vi "FMDemo2 (SubVI).vi"(9 "Numeric":dbl, 10 "Array":cdb[](array[numeric]), 11 "Sample Rate":dbl) -> (3 "Decimated Array":dbl[](array[numeric]))   [LabVIEW 2013]
uses:
  <vilib>/Analysis/3filter.llb/Filter Passband Type.ctl
  <vilib>/Analysis/3filter.llb/Butterworth Filter (CDB).vi
  <vilib>/Analysis/2dsp.llb/Decimate (continuous, DBL).vi
  <vilib>/Analysis/NI_AALBase.lvlib
  <vilib>/Analysis/NI_AALPro.lvlib
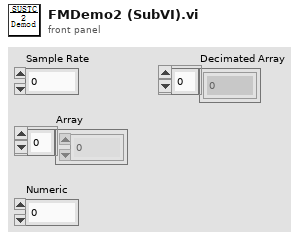
[diagram p1: front panel]
types:
  T1 = typedef "NI_AALBase.lvlib/Filter Passband Type.ctl" = enum32{"Lowpass", "Highpass", "Bandpass", "Bandstop"}
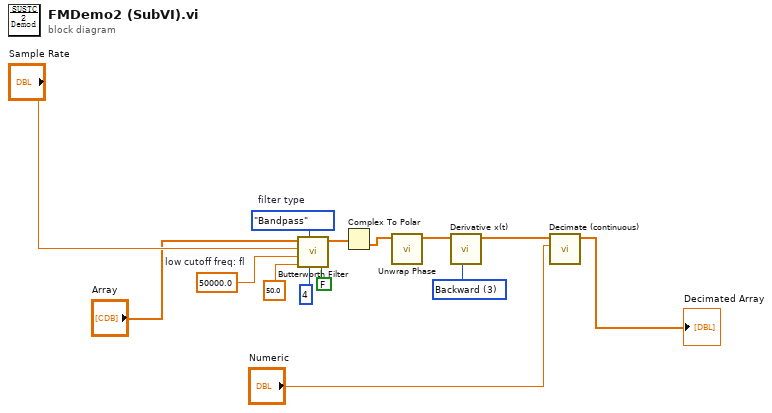
[diagram p0: block diagram]
diagram:
  w3 = u16 3 items=["2nd Order Central", "4th Order Central", "Forward", "Backward"] ("method")
  w2 = Filter_Passband_Type."Bandpass"  # filter type
  w5 = 50000.0  # low cutoff freq: fl
  n1 = call-poly <vilib>:"Butterworth Filter.vi"("init/cont (init:F)"=FALSE, "order"=4, "filter type"=w2, "low cutoff freq: fl"=50.0, "high cutoff freq: fh"=w5, "sampling freq: fs"="Sample Rate", "X"="Array") -> ("Filtered X"=w12:cdb[])  [unwired: 1 in, 1 out]
  n2 = Complex To Polar(r * e^(i*theta)=w12) -> (theta=w7:dbl[])  [unwired: 1 out]
  n3 = call <vilib>:"Unwrap Phase.vi"("Phase"=w7) -> ("Unwrapped Phase"=w4:dbl[])  [unwired: 9 in, 1 out]
  n4 = call <vilib>:"Derivative x(t).vi"("method"=w3, "X"=w4) -> ("dX/dt"=w8:dbl[])  [unwired: 8 in, 1 out]
  n5 = call-poly <vilib>:"Decimate (continuous).vi"("decimating factor"="Numeric", "X"=w8) -> ("Decimated Array"=→"Decimated Array":dbl[])  [unwired: 8 in, 1 out]
